vi "Read Slot Programming Modes Supported.vi"(8 "error in (no error)":errorcluster, 11 "RSI Module in":refnum<class "RSI Module.lvclass">) -> (0 "error out":errorcluster, 2 "Slot Programming Modes Supported":u8, 3 "RSI Module out":refnum<class "RSI Module.lvclass">)   [LabVIEW 2017, in "Modules.lvlib" / "RSI Module.lvclass"]
uses:
  RSI Module.lvclass
  RSI Module.lvclass/RSI Module.ctl
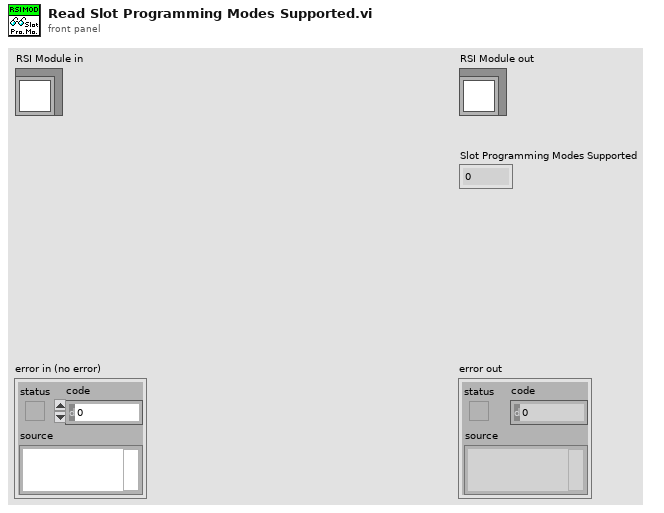
[diagram p1: front panel]
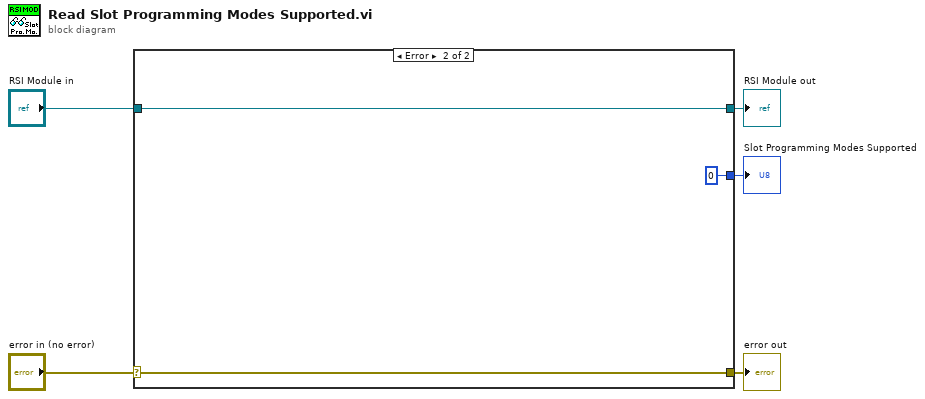
[diagram p0: block diagram]
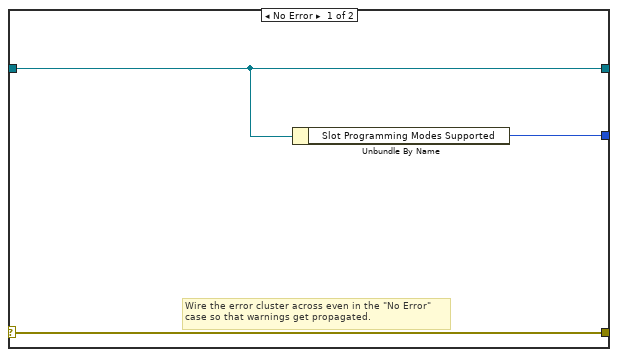
[diagram p2: hidden frame]
diagram:
  n1 = case shown="Error" "error in (no error)" {
    selector: "error in (no error)" -> [w8 w11]
    tunnel: [w8 w11] -> w4
    tunnel: [w7 w10] -> w2
    tunnel: "RSI Module in" -> [w7 w10]
    tunnel: [w6 u8 0 ("Slot Programming Modes Supported")] -> w1
    frame No Error {
      # "Wire the error cluster across even in the \"No Error\"\ncase so that warnings get propagated."
      n2 = Unbundle By Name(w7) -> ("Slot Programming Modes Supported"=w6:u8)
    }
    frame Error {
    }
  }
  "error out" <- w4
  "RSI Module out" <- w2
  "Slot Programming Modes Supported" <- w1
